vi "SR Doppler.vi"() -> ()   [LabVIEW 2012]
uses:
  user.lib/SpectralRadar.llb/Scan Pattern.lvclass
  user.lib/SpectralRadar.llb/Probe.lvclass
  user.lib/SpectralRadar.llb/Coloring.lvclass
  user.lib/SpectralRadar.llb/Colorscheme Selection.ctl
  user.lib/SpectralRadar.llb/Doppler Flag.ctl
  user.lib/SpectralRadar.llb/Coloring Byteorder.ctl
  <vilib>/Utility/error.llb/DialogType.ctl
  user.lib/SpectralRadar.llb/Calibration Selection.ctl
  user.lib/SpectralRadar.llb/Probe Parameter Int Selection.ctl
  user.lib/SpectralRadar.llb/Processing Parameter Int Selection.ctl
  user.lib/SpectralRadar.llb/Doppler Property Int.ctl
  user.lib/SpectralRadar.llb/set Complex Scan Output.vi
  user.lib/SpectralRadar.llb/display Data 2D.vi
  user.lib/SpectralRadar.llb/Doppler Processing.lvclass
  user.lib/SpectralRadar.llb/LabVIEW Helper.lvlib
  user.lib/SpectralRadar.llb/OCT Device.lvclass
  user.lib/SpectralRadar.llb/Processing.lvclass
  user.lib/SpectralRadar.llb/FullRange.lvclass
  user.lib/SpectralRadar.llb/Settings.lvclass
  user.lib/SpectralRadar.llb/FileSelection.lvlib
  user.lib/SpectralRadar.llb/Raw Data.lvclass
  user.lib/SpectralRadar.llb/Data.lvclass
  user.lib/SpectralRadar.llb/Colored Data.lvclass
  user.lib/SpectralRadar.llb/Complex Data.lvclass
panel:
  in  "Averaging Z":i32=1 min=1 max=20 step=1
  in  "Averaging X":i32=2 min=2 max=20 step=1
  out "Phase Graph":dbl[][](graph)
  out "Amplitude Graph":dbl[][](graph)
  in  "Absolute Phase Threshold":sgl=0.2
  in  "Signal Threshold [dB]":sgl
  out "Coloring":refnum<class "Coloring.lvclass">
  out "GalvoControl":refnum<class "Probe.lvclass">
  out "Scan Pattern":refnum<class "Scan Pattern.lvclass">
  out "AutoSafe":bool
  in  "Binning":i32(slide)=1 caption="Quality" min=1 max=200 step=1 scale=1.0..200.0
  in  "Options":bool
  in  "Window":T1(ring)
  in  "Palette":T2(ring)
  in  "ShowVideoImage":bool caption="Show Video Image"
  out "StreamingPath":path
  out "Image":T3(plugin-control)
  out "Frame Rate":dbl=6.134969234466553 format="%#_3g"
  in  "RunMeasurement":bool
  out "StopIndicator":bool
  in  "Brightness":sgl(slide)=0.5272727 caption="Sharpness" min=0 max=1 step=0.01 scale=0.0..1.0
  in  "Contrast":sgl(slide)=0.53333336 caption="Sharpness" min=0 max=1 step=0.01 scale=0.0..1.0
  in  "Saturation":sgl(slide)=0.5212121 caption="Sharpness" min=0 max=1 step=0.01 scale=0.0..1.0
  out "Spacing Z":dbl=2.0 min=1.0 max=500.0 step=1.0 format="%-#2_3f"
  in  "LowerBScanBorder":dbl=0.972000002861023 min=0.75 max=5.12 step=0.1 format="%.2f"
  in  "UpperBScanBorder":dbl min=0.0 max=0.5 step=0.10000000149011612 format="%.2f"
  out "Reference Intensity":sgl(slide) max=140000 scale=0.0..1.0
  out "Next File Name":path=path "D:/OCTData"
  in  "Set Path":bool
  in  "Recallibrate":bool
  in  "Range X [mm]":dbl=2.0 caption="Bereich [mm]" min=0.0 max=10.0 step=0.5 format="%_3f"
  out "Spacing X [µm]":dbl=2.0 min=1.0 max=500.0 step=1.0 format="%#_3g"
  in  "Columns":i32=1000 min=50 max=2500 step=1
  in  "Index of Refraction":dbl=1.0 min=1.0 max=5.0 step=0.10000000149011612 format="%.3f"
  in  "QuitApp":bool
  in  "Boundries":cluster{sgl, sgl}(slide)={76.65738, 42.00557} scale=-20.0..150.0
  out "B-Scan":sgl[][](graph)
  # "Version 5.1"
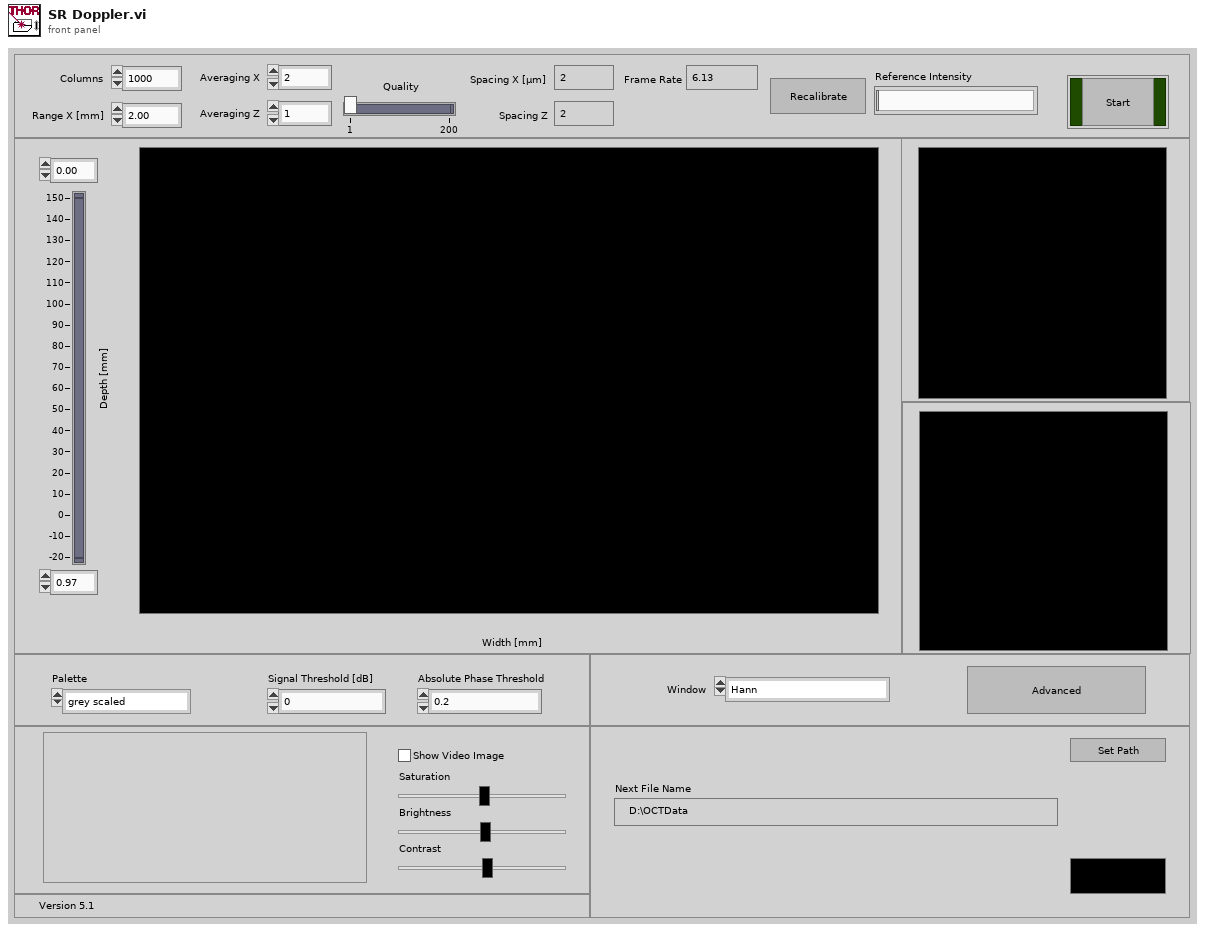
[diagram p1: front panel]
types:
  T1 = enum16{"Hann", "Hamming", "Gauss", "Tapered Cosine", "Blackman", "4 Term B-Harris"}
  T2 = enum16{"grey scaled", "grey scaled (inverted)", "color coded", "orange-black", "red-black"}
  T3 = typedef "IMAQ Image.ctl" = refnum<image>
  T4 = typedef "Coloring.lvclass/Coloring Byteorder.ctl" = enum16{"RGBA32", "BGRA32", "ARGB32", ""}
  T5 = typedef "Doppler Processing.lvclass/Doppler Flag.ctl" = enum16{"Doppler Velocity Scaling"}
  T6 = typedef "Coloring.lvclass/Colorscheme Selection.ctl" = enum16{"Black And White", "Inverted Black And White", "Color", "Black and Orange", "Black and Red", "Doppler Phase Coloring"}
  T7 = enum16{"Full Well Capacity", "z Spacing", "z Range", "Dynamc Range Min [dB]", "Dynamic Range Low [dB]", "Dynamic Range High [dB]", "Dynamic Range Max [dB]"}
  T8 = typedef "Processing.lvclass/Calibration Selection.ctl" = enum16{"Offset Errors", "Apodization Spectrum", "Apodization Vector", "Dispersion", "Chirp", "Extended Adjust", "Fixed Pattern"}
  T9 = typedef "Processing.lvclass/Processing Parameter Int Selection.ctl" = enum32{"Spectrum Averaging", "A-Scan Averaging", "B-Scan Averaging", "Zero Padding", "Number of Threads", "Fourier Averaging"}
  T10 = typedef "Probe.lvclass/Probe Parameter Int Selection.ctl" = enum16{"Apodization Cycles", "Oversampling", "Oversampling Slow Axis", "Speckle Reduction"}
  T11 = typedef "Doppler Processing.lvclass/Doppler Property Int.ctl" = enum16{"Doppler Averaging 1", "Doppler Averaging 2"}
  T12 = enum16{"Asynchronous Continuous", "Asynchronous Finite", "Synchronous"}
  T13 = typedef "Image Type" = u32
  T14 = typedef "DialogType.ctl" = u16
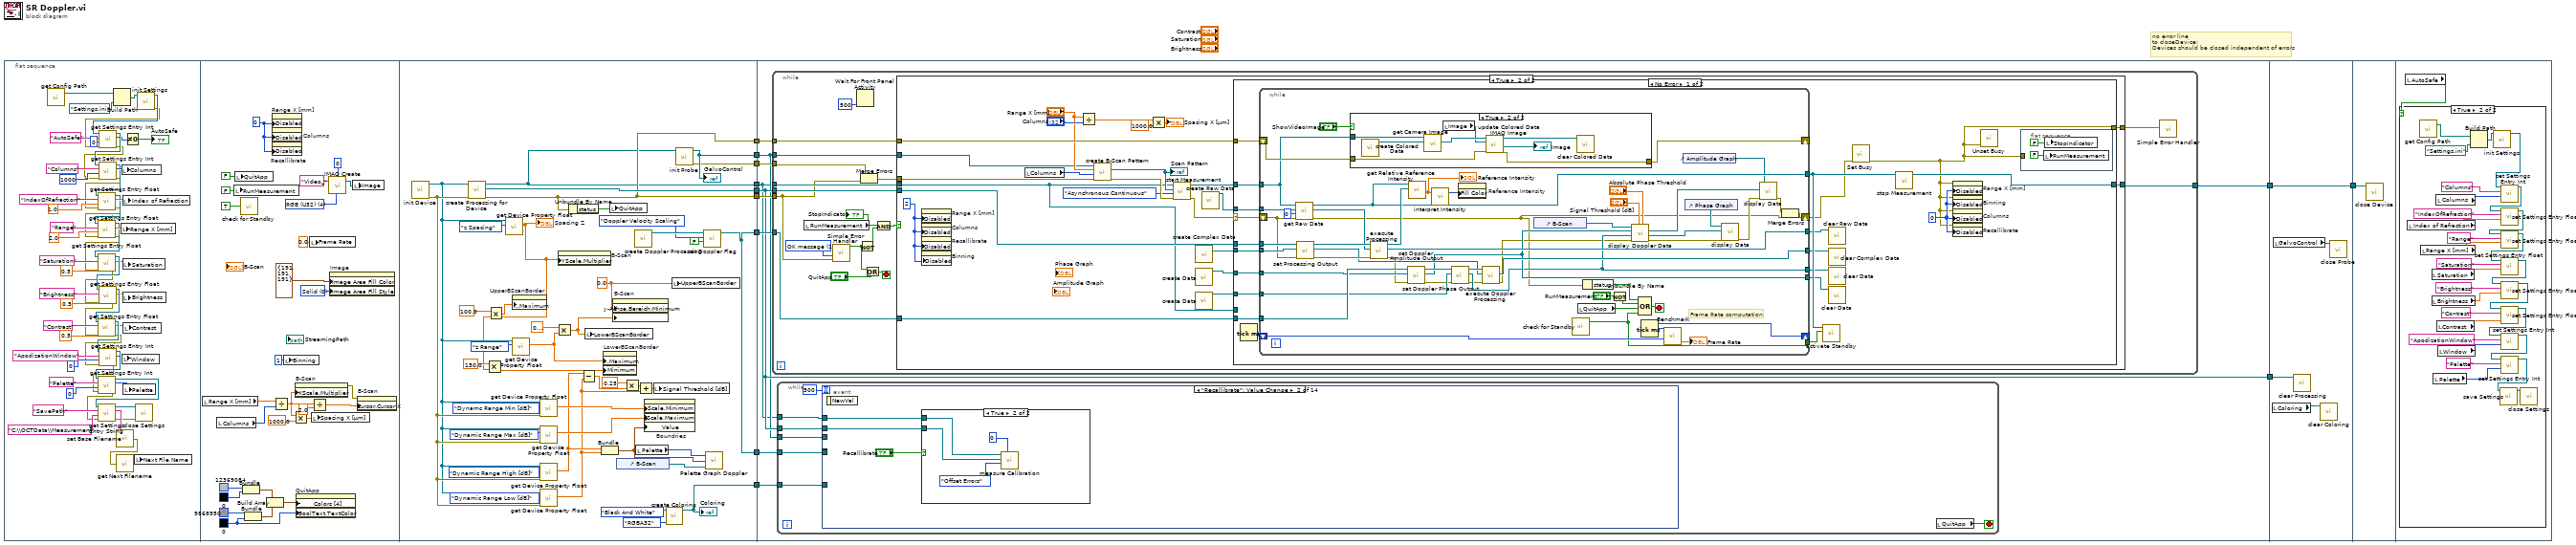
[diagram p0: block diagram]
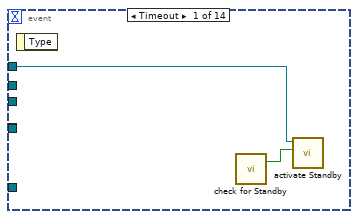
[diagram p2: hidden frame]
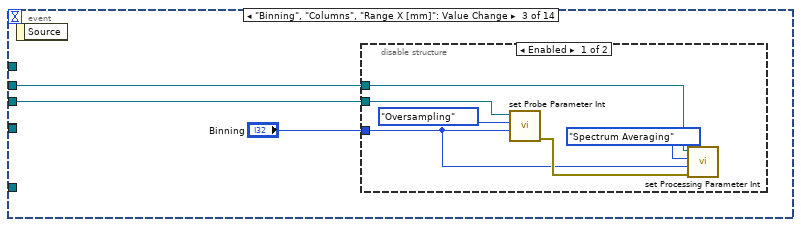
[diagram p4: hidden frame]
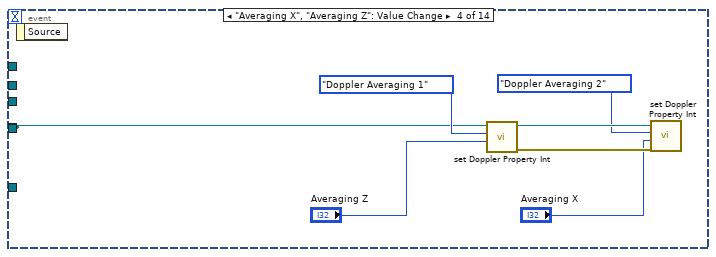
[diagram p6: hidden frame]
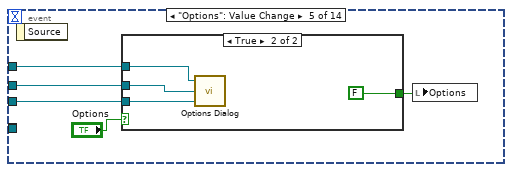
[diagram p7: hidden frame]
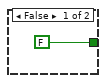
[diagram p8: hidden frame]
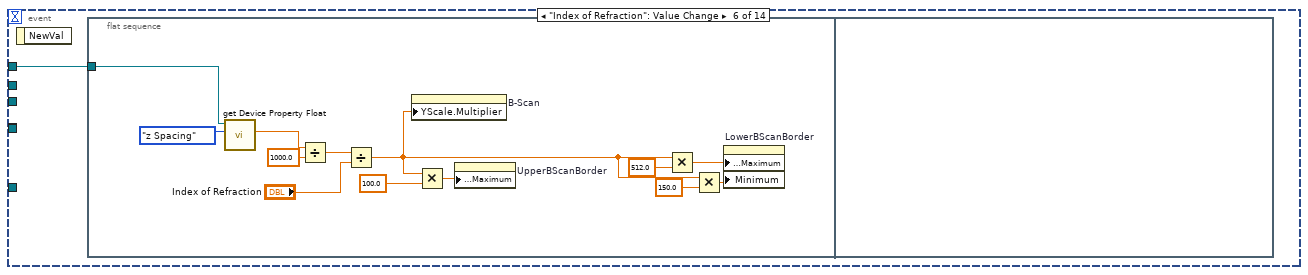
[diagram p9: hidden frame]
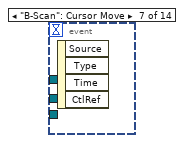
[diagram p10: hidden frame]
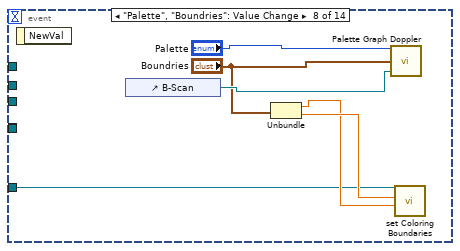
[diagram p11: hidden frame]
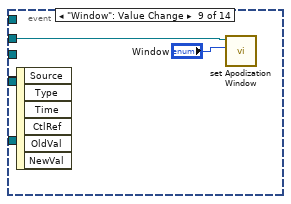
[diagram p12: hidden frame]
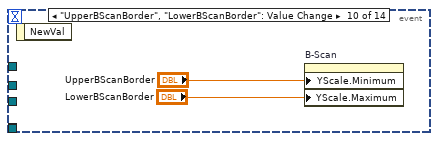
[diagram p13: hidden frame]
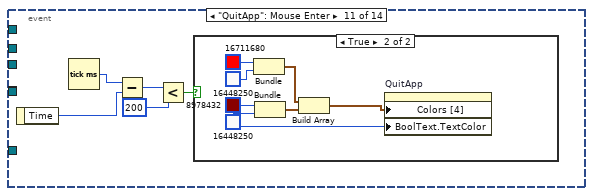
[diagram p14: hidden frame]
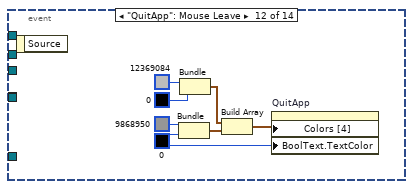
[diagram p16: hidden frame]
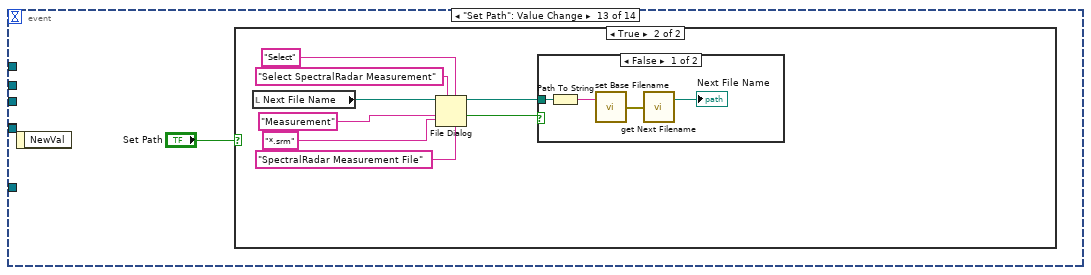
[diagram p17: hidden frame]
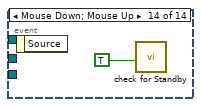
[diagram p20: hidden frame]
diagram:
  # "no error line\nto closeDevice:\nDevices should be closed independent of errors"
  n1 = flat-sequence {
    tunnel: [w109] -> w12
    tunnel: [w116] -> w9
    tunnel: [w128] -> w8
    tunnel: [w131] -> w6
    tunnel: [w116] -> w5
    tunnel: [w129] -> w4
    tunnel: [w113] -> w3
    tunnel: [w101] -> w2
    tunnel: [w101] -> w1
    tunnel: w12 -> [w141]
    tunnel: [w148] -> w10
    tunnel: w9 -> [w147]
    tunnel: w8 -> [w143]
    tunnel: [w143] -> w7
    tunnel: w6 -> [w142]
    tunnel: w5 -> [w146]
    tunnel: w4 -> [w145]
    tunnel: w3 -> [w139]
    tunnel: w2 -> [w144]
    tunnel: w1 -> [w140]
    tunnel: [w382] -> w11
    tunnel: w10 -> [w382]
    tunnel: w7 -> [w381]
    tunnel: w11 -> [w383]
    frame #0 {
      n2 = call "get Config Path.vi"() -> ("Path"=w24:path)  [unwired: 1 in, 1 out]
      n3 = Build Path(base path=w24, name or relative path=path "Settings.ini" ("Relative \"SpectralRadar.ini\" Path")) -> (appended path=w69:path)
      n4 = call "init Settings.vi"("Path to settings file"=w69) -> ("error out"=w23:errorcluster, "Settings"=w56:refnum<class "Settings.lvclass">)  [unwired: 5 in]
      n5 = call "get Settings Entry Int.vi"("error in (no error)"=w23, "Default Value"=0, "Node Name"="AutoSafe", "Settings"=w56) -> ("error out"=w21:errorcluster, "Value"=w53:i32, "Settings"=w57:refnum<class "Settings.lvclass">)  [unwired: 1 in]
      n6 = call "get Settings Entry Int.vi"("error in (no error)"=w21, "Default Value"=1000, "Node Name"="Columns", "Settings"=w57) -> ("error out"=w20:errorcluster, "Value"=w67:i32, "Settings"=w59:refnum<class "Settings.lvclass">)  [unwired: 1 in]
      n7 = call "get Settings Entry Float.vi"("error in (no error)"=w20, "Default Value"=1.0, "Node Name"="IndexOfRefraction", "Settings"=w59) -> ("error out"=w19:errorcluster, "Value"=w63:dbl, "Settings"=w58:refnum<class "Settings.lvclass">)  [unwired: 1 in]
      n8 = call "get Settings Entry Float.vi"("error in (no error)"=w19, "Default Value"=2.0, "Node Name"="Range", "Settings"=w58) -> ("error out"=w18:errorcluster, "Value"=w60:dbl, "Settings"=w49:refnum<class "Settings.lvclass">)  [unwired: 1 in]
      n9 = call "get Settings Entry Float.vi"("error in (no error)"=w18, "Default Value"=0.5, "Node Name"="Saturation", "Settings"=w49) -> ("error out"=w17:errorcluster, "Value"=w34:dbl, "Settings"=w46:refnum<class "Settings.lvclass">)  [unwired: 1 in]
      n10 = call "get Settings Entry Float.vi"("error in (no error)"=w17, "Default Value"=0.5, "Node Name"="Brightness", "Settings"=w46) -> ("error out"=w16:errorcluster, "Value"=w33:dbl, "Settings"=w39:refnum<class "Settings.lvclass">)  [unwired: 1 in]
      n11 = call "get Settings Entry Float.vi"("error in (no error)"=w16, "Default Value"=0.5, "Node Name"="Contrast", "Settings"=w39) -> ("error out"=w15:errorcluster, "Value"=w32:dbl, "Settings"=w38:refnum<class "Settings.lvclass">)  [unwired: 1 in]
      n12 = call "get Settings Entry Int.vi"("error in (no error)"=w15, "Default Value"=0, "Node Name"="ApodizationWindow", "Settings"=w38) -> ("error out"=w14:errorcluster, "Value"=w36:i32, "Settings"=w37:refnum<class "Settings.lvclass">)  [unwired: 1 in]
      n13 = call "get Settings Entry Int.vi"("error in (no error)"=w14, "Default Value"=0, "Node Name"="Palette", "Settings"=w37) -> ("error out"=w13:errorcluster, "Value"=w35:i32, "Settings"=w30:refnum<class "Settings.lvclass">)  [unwired: 1 in]
      n14 = call "get Settings Entry String.vi"("error in (no error)"=w13, "Default Value"="C:\\OCTData\\Measurement", "Node Name"="SavePath", "Settings"=w30) -> ("error out"=w22:errorcluster, "Value"=w27:string, "Settings"=w29:refnum<class "Settings.lvclass">)  [unwired: 1 in]
      n15 = call "set Base Filename.vi"("Base"=w27) -> ("error out"=w26:errorcluster)  [unwired: 1 in]
      n16 = call "get Next Filename.vi"("error in (no error)"=w26) -> ("Next File Name"=w25:path)  [unwired: 1 out]
      n17 = local write "Range X [mm]"(w60) -> ()
      n18 = local write "Columns"(w67) -> ()
      n19 = local write "Window"(w36) -> ()
      n20 = local write "Index of Refraction"(w63) -> ()
      n21 = local write "Saturation"(w34) -> ()
      n22 = local write "Brightness"(w33) -> ()
      n23 = local write "Contrast"(w32) -> ()
      n24 = local write "Palette"(w35) -> ()
      n25 = Not Equal To 0?(x=w53) -> (x != 0?=→"AutoSafe":bool)
      n26 = local write "Next File Name"(w25) -> ()
      n27 = call "close Settings.vi"("error in (no error)"=w22, "Settings"=w29) -> ()  [unwired: 5 in, 1 out]
    }
    frame #1 {
      w73 = T13 4 items=["Grayscale (U8)", "Grayscale (I16)", "Grayscale (SGL)", "Complex (CSG)", "RGB (U32)", "HSL (U32)", "RGB (U64)", "Grayscale (U16)"] ("Image Type")
      w78 = u32 0 items=["Default"=3, "Solid"=0, "Hatch"=2] ("Image Area:Background:Fill Style")
      w93 = u32 0
      w97 = u8 0 ("Deaktiviert")
      n28 = local read "Range X [mm]"() -> (w85:dbl)
      n29 = local read "Columns"() -> (w80:i32)
      n30 = local write "RunMeasurement"(FALSE ("s/t")) -> ()
      n31 = local write "QuitApp"(FALSE ("QuitApp")) -> ()
      n32 = call "check for Standby.vi"("ResetTimer"=TRUE) -> ()  [unwired: 2 out]
      n33 = Bundle(u32 12369084, u32 0) -> (w90:cluster{u32, u32})  [unwired: 1 in]
      n34 = Bundle(u32 9868950, w93) -> (w91:cluster{u32, u32})  [unwired: 1 in]
      n35 = Build Array(w90, w91) -> (w92:cluster{u32, u32}[])
      n36 = property on="Range X [mm]" class="DigNum (strict)"("Disabled"=w97) -> ()  [unwired: 2 in, 2 out]
      n37 = property on="Columns" class="DigNum (strict)"("Disabled"=w97) -> ()  [unwired: 2 in, 2 out]
      n38 = property on="Recallibrate" class="Bool"("Disabled"=w97) -> ()  [unwired: 2 in, 2 out]
      n39 = Divide(x=w85, y=w80) -> (x/y=w83:dbl)
      n40 = local write "Binning"(1 ("Binning")) -> ()
      n41 = Multiply(x=w83, y=1000.0) -> (x*y=w81:dbl)
      n42 = property on="B-Scan" class="IntGraph (strict)"("XScale.Multiplier"=w83) -> (error out=w86:errorcluster)  [unwired: 2 in, 1 out]
      n43 = property on="QuitApp" class="Bool (strict)"("Colors [4]"=w92, "BoolText.TextColor"=w93) -> ()  [unwired: 2 in, 2 out]
      n44 = local write "Frame Rate"(0.0 ("Frame Rate")) -> ()
      n45 = Divide(x=w83, y=2.0) -> (x/y=w82:dbl)
      n46 = local write "Spacing X [µm]"(w81) -> ()
      n47 = call "IMAQ Create"("Border Size"=0, "Image Name"="Video_", "Image Type"=w73) -> ("New Image"=w71:T3)  [unwired: 2 in, 1 out]
      n48 = property on="Image" class="ImageControl"("Image Area Fill Color"=cluster{"Red":u8, "Green":u8, "Blue":u8} {"Red"=191, "Green"=191, "Blue"=191} ("Image Area:Background:Fill Color"), "Image Area Fill Style"=w78) -> ()  [unwired: 2 in, 2 out]
      n49 = local write "Image"(w71) -> ()
      n50 = property on="B-Scan" class="IntGraph (strict)"(error in=w86, "Cursor.Cursor X"=w82) -> ()  [unwired: 1 in, 2 out]
    }
    frame #2 {
      w133 = 0.0 ("y")
      n51 = call "init Device.vi"() -> ("error out"=w127:errorcluster, "OCTDevice"=w120:refnum<class "OCT Device.lvclass">)  [unwired: 6 in]
      n52 = call "create Processing for Device.vi"("error in (no error)"=w127, "OCTDevice"=w120) -> ("error out"=w116:errorcluster, "Processing"=w128:refnum<class "Processing.lvclass">, "OCTDevice"=w109:refnum<class "OCT Device.lvclass">)  [unwired: 3 in]
      n53 = call "get Device Property Float.vi"("Device Property Float Selection"=T7."z Spacing", "OCTDevice"=w120) -> ("Value"=w115:dbl)  [unwired: 3 in, 2 out]
      "Spacing Z" <- w115
      n54 = Multiply(x=150.0, y=w115) -> (x*y=w135:dbl)
      n55 = Multiply(x=100.0, y=w115) -> (x*y=w138:dbl)
      n56 = property on="UpperBScanBorder" class="DigNum (strict)"("Wertebereich:Maximum"=w138) -> ()  [unwired: 2 in, 2 out]
      n57 = call "get Device Property Float.vi"("Device Property Float Selection"=T7."z Range", "OCTDevice"=w120) -> ("Value"=w118:dbl)  [unwired: 3 in, 2 out]
      n58 = call "get Device Property Float.vi"("error in (no error)"=w127, "Device Property Float Selection"=T7."Dynamc Range Min [dB]", "OCTDevice"=w120) -> ("Value"=w126:dbl)  [unwired: 2 in, 2 out]
      n59 = call "get Device Property Float.vi"("error in (no error)"=w127, "Device Property Float Selection"=T7."Dynamic Range Max [dB]", "OCTDevice"=w120) -> ("Value"=w125:dbl)  [unwired: 2 in, 2 out]
      n60 = call "get Device Property Float.vi"("error in (no error)"=w127, "Device Property Float Selection"=T7."Dynamic Range High [dB]", "OCTDevice"=w120) -> ("Value"=w107:dbl)  [unwired: 2 in, 2 out]
      n61 = call "get Device Property Float.vi"("error in (no error)"=w127, "Device Property Float Selection"=T7."Dynamic Range Low [dB]", "OCTDevice"=w120) -> ("Value"=w106:dbl)  [unwired: 2 in, 2 out]
      n62 = Multiply(x=0.800000011920929, y=w118) -> (x*y=w132:dbl)
      n63 = property on="B-Scan" class="IntGraph (strict)"("YScale.Multiplier"=w115) -> ()  [unwired: 2 in, 2 out]
      n64 = Unbundle By Name(w116) -> ("status"=w130:bool)
      n65 = Subtract(x=w107, y=w106) -> (x-y=w104:dbl)
      n66 = local write "LowerBScanBorder"(w132) -> ()
      n67 = Bundle("Value"=w107, "Value"=w106) -> (w112:cluster{"Value":dbl, "Value":dbl})  [unwired: 1 in]
      n68 = property on="LowerBScanBorder" class="DigNum (strict)"("Wertebereich:Maximum"=w118, "Minimum"=w135) -> ()  [unwired: 2 in, 2 out]
      n69 = local write "QuitApp"(w130) -> ()
      n70 = property on="B-Scan" class="IntGraph (strict)"("y-Achse.Bereich:Minimum"=w133, "y-Achse.Bereich:Maximum"=w132) -> ()  [unwired: 2 in, 2 out]
      n71 = control-ref of="B-Scan"() -> (w110:refnum<vi>)
      n72 = Multiply(x=0.25, y=w104) -> (x*y=w105:dbl)
      n73 = call "create Doppler Processing.vi"() -> ("Doppler Processing"=w102:refnum<class "Doppler Processing.lvclass">)  [unwired: 6 in, 1 out]
      n74 = local read "Palette"() -> (w111:T2)
      n75 = Add(x=w105, y=w106) -> (x+y=w108:dbl)
      n76 = property on="Boundries" class="Slide (strict)"("Scale.Minimum"=w126, "Scale.Maximum"=w125, "Value"=w112) -> ()  [unwired: 2 in, 2 out]
      n77 = local write "Signal Threshold [dB]"(w108) -> ()
      n78 = call "create Coloring.vi"("Color Byte Order"=Coloring_Byteorder."RGBA32", "Color Table Selection"=Colorscheme_Selection."Black And White") -> ("Coloring"=w113:refnum<class "Coloring.lvclass">)  [unwired: 4 in, 1 out]
      "Coloring" <- w113
      n79 = local write "UpperBScanBorder"(w133) -> ()
      n80 = call "init Probe.vi"("OCT Device"=w109) -> ("error out"=w129:errorcluster, "GalvoControl"=w131:refnum<class "Probe.lvclass">)  [unwired: 5 in]
      "GalvoControl" <- w131
      n81 = call "set Doppler Flag.vi"("Boolean"=FALSE, "Doppler Flag"=Doppler_Flag."Doppler Velocity Scaling", "DopplerProcessing in"=w102) -> ("DopplerProcessing out"=w101:refnum<class "Doppler Processing.lvclass">)  [unwired: 3 in, 1 out]
      n82 = call "Palette Graph Doppler.vi"("Reference to the B-scan Graph"=w110, "Boundaries"=w112, "Palette"=w111) -> ()
    }
    frame #3 {
      n83 = while {
        tunnel: w141 -> [w261]
        tunnel: [w260] -> w148
        tunnel: w147 -> [w259]
        tunnel: w143 -> [w258]
        tunnel: w142 -> [w257]
        tunnel: w146 -> [w256]
        tunnel: w145 -> [w250]
        tunnel: w144 -> [w248]
        stop <- w263 stop-if-true
        w249 = T14 1 items=["no dialog", "OK message", "continue or stop message", "OK message + warnings", "continue/stop + warnings"] ("type of dialog (OK msg:1)")
        n84 = local read "RunMeasurement"() -> (w254:bool)
        "StopIndicator" <- w254
        n85 = call <vilib>:"Simple Error Handler.vi"("type of dialog (OK msg:1)"=w249, "error in (no error)"=w256) -> ("error?"=w253:bool)  [unwired: 3 in, 4 out]
        n86 = Wait For Front Panel Activity(1:500 ("Timeout in ms (-1 kein Timeout)")) -> ()  [unwired: 2 in, 1 out]
        n87 = Not(x=w253) -> (.not. x?=w252:bool)
        n88 = Merge Errors(w250, w256) -> (w251:errorcluster)
        n89 = Or(x=w253, y="QuitApp") -> (x .or. y?=w263:bool)
        n90 = And(x=w254, y=w252) -> (x .and. y?=w255:bool)
        n91 = case shown="True" w255 {
          tunnel: [w267 w291] -> w265
          tunnel: w251 -> [w267 w268]
          tunnel: w261 -> [w266 w274]
          tunnel: [w266 w285] -> w260
          tunnel: w259 -> [_ w284]
          tunnel: w258 -> [_ w278]
          tunnel: w257 -> [_ w280]
          tunnel: w248 -> [_ w269]
          frame False {
          }
          frame True {
            w279 = u8 2 ("Deaktiviert")
            n92 = property on="Range X [mm]" class="DigNum (strict)"("Disabled"=w279) -> ()  [unwired: 2 in, 2 out]
            n93 = property on="Columns" class="DigNum (strict)"("Disabled"=w279) -> ()  [unwired: 2 in, 2 out]
            n94 = property on="Recallibrate" class="Bool"("Disabled"=w279) -> ()  [unwired: 2 in, 2 out]
            n95 = property on="Binning" class="Slide (strict)"("Disabled"=w279) -> ()  [unwired: 2 in, 2 out]
            n96 = local read "Columns"() -> (w282:i32)
            n97 = Divide(x="Range X [mm]", y="Columns") -> (x/y=w289:dbl)
            n98 = call "create B-Scan Pattern.vi"("error in (no error)"=w268, "AScans"=w282, "Range"="Range X [mm]", "Probe"=w280) -> ("error out"=w281:errorcluster, "Scan Pattern"=w277:refnum<class "Scan Pattern.lvclass">)  [unwired: 2 in, 1 out]
            "Scan Pattern" <- w277
            n99 = Multiply(x=w289, y=1000.0) -> (x*y=→"Spacing X [µm]":dbl)
            n100 = call "start Measurement.vi"("error in (no error)"=w281, "Acquisition Type"=T12."Asynchronous Continuous", "Scan Pattern"=w277, "OCTDevice"=w274) -> ("error out"=w275:errorcluster, "OCTDevice"=w290:refnum<class "OCT Device.lvclass">)  [unwired: 1 in, 1 out]
            n101 = call "create Data.vi"() -> ("Data"=w271:refnum<class "Data.lvclass">)  [unwired: 6 in, 1 out]
            n102 = call "create Data.vi"() -> ("Data"=w270:refnum<class "Data.lvclass">)  [unwired: 6 in, 1 out]
            n103 = call "create Complex Data.vi"() -> ("Complex Data"=w272:refnum<class "Complex Data.lvclass">)  [unwired: 2 in, 1 out]
            n104 = call "create Raw Data.vi"() -> ("Raw Data"=w276:refnum<class "Raw Data.lvclass">)  [unwired: 6 in, 1 out]
            n105 = case shown="No Error" w275 {
              selector: w275 -> [w302 w378]
              tunnel: [w303 _] -> w291
              tunnel: w284 -> [w311 _]
              tunnel: w290 -> [w310 w375]
              tunnel: [w309 w374] -> w285
              tunnel: w278 -> [w305 _]
              tunnel: w276 -> [w301 _]
              tunnel: w274 -> [_ _]
              tunnel: w272 -> [w298 _]
              tunnel: w271 -> [w297 _]
              tunnel: w270 -> [w296 _]
              tunnel: w269 -> [w295 _]
              frame No Error {
                w304 = u8 0 ("Deaktiviert")
                n106 = Tick Count (ms)() -> (millisecond timer value=w307:u32)
                n107 = while {
                  shift-right: [w362] -> _
                  shift-left: w307 -> [w360]
                  tunnel: w310 -> [w353]
                  tunnel: [w351] -> w306
                  tunnel: [w335] -> w308
                  tunnel: w305 -> [w349]
                  shift-right: [w354] -> _
                  shift-left: w311 -> [w364]
                  shift-right: [w318] -> w300
                  shift-left: w302 -> [w321]
                  tunnel: w301 -> [w352]
                  tunnel: [w343] -> w299
                  tunnel: w298 -> [w342]
                  tunnel: w297 -> [w340]
                  tunnel: w296 -> [w338]
                  tunnel: w295 -> [w341]
                  tunnel: [w331] -> w294
                  tunnel: [w332] -> w293
                  tunnel: [w334] -> w292
                  stop <- w358 stop-if-true
                  # "Frame Rate computation"
                  n108 = call "get Raw Data.vi"("error in (no error)"=w321, "Camera Index"=0, "RawData in"=w352, "OCTDevice in"=w353) -> ("error out"=w319:errorcluster, "RawData out"=w347:refnum<class "Raw Data.lvclass">, "OCTDevice out"=w335:refnum<class "OCT Device.lvclass">)  [unwired: 1 in]
                  n109 = call-poly "set Processing Output.vi"("error in (no error)"=w321, "Complex Data in"=w342, "Processing"=w349) -> ("error out"=w346:errorcluster, "Complex Data out"=w336:refnum<class "Complex Data.lvclass">, "Processing"=w348:refnum<class "Processing.lvclass">)  [unwired: 2 in]
                  n110 = case shown="True" "ShowVideoImage" {
                    tunnel: w353 -> [_ w373]
                    tunnel: w364 -> [w365 w370]
                    tunnel: [w365 w369] -> w354
                    frame False {
                    }
                    frame True {
                      n111 = call "create Colored Data.vi"() -> ("Colored Data"=w372:refnum<class "Colored Data.lvclass">)  [unwired: 6 in, 1 out]
                      n112 = call "get Camera Image.vi"("Colored Data in"=w372, "OCTDevice in"=w373) -> ("Colored Data out"=w371:refnum<class "Colored Data.lvclass">)  [unwired: 5 in, 2 out]
                      n113 = local read "Image"() -> (w367:T3)
                      n114 = call "update Colored Data IMAQ Image.vi"("error in (no error)"=w370, "Image in"=w367, "Colored Data"=w371) -> ("error out"=w369:errorcluster, "Image out"=→"Image":T3, "Colored Data"=w366:refnum<class "Colored Data.lvclass">)  [unwired: 2 in]
                      n115 = call "clear Colored Data.vi"("Colored Data"=w366) -> ()  [unwired: 6 in, 1 out]
                    }
                  }
                  n116 = call "execute Processing.vi"("error in (no error)"=w346, "Raw Data"=w347, "Processing"=w348) -> ("error out"=w317:errorcluster, "Raw Data"=w343:refnum<class "Raw Data.lvclass">, "Processing"=w345:refnum<class "Processing.lvclass">)  [unwired: 2 in]
                  n117 = call "set Doppler Amplitude Output.vi"("error in (no error)"=w317, "Data in"=w340, "DopplerProcessing in"=w341) -> ("error out"=w316:errorcluster, "Data out"=w332:refnum<class "Data.lvclass">, "DopplerProcessing out"=w339:refnum<class "Doppler Processing.lvclass">)  [unwired: 2 in]
                  n118 = call "get Relative Reference Intensity.vi"("Processing"=w345, "OCTDevice"=w335) -> ("Relative Reference Intensity"=w344:dbl)  [unwired: 2 in, 3 out]
                  "Reference Intensity" <- w344
                  n119 = call "interpret Intensity.vi"("Intensity"=w344) -> ("Color"=w356:u32)  [unwired: 1 in, 1 out]
                  n120 = call "set Doppler Phase Output.vi"("error in (no error)"=w316, "Data in"=w338, "DopplerProcessing in"=w339) -> ("error out"=w315:errorcluster, "Data out"=w331:refnum<class "Data.lvclass">, "DopplerProcessing out"=w337:refnum<class "Doppler Processing.lvclass">)  [unwired: 2 in]
                  n121 = property on="Reference Intensity" class="Slide (strict)"("Fill Color"=w356) -> ()  [unwired: 2 in, 2 out]
                  n122 = call "execute Doppler Processing.vi"("error in (no error)"=w315, "Complex Data in"=w336, "DopplerProcessing in"=w337) -> ("error out"=w330:errorcluster, "Complex Data out"=w334:refnum<class "Complex Data.lvclass">)  [unwired: 2 in, 1 out]
                  n123 = control-ref of="B-Scan"() -> (w333:refnum<vi>)
                  n124 = call "check for Standby.vi"() -> ("TimeOut"=w351:bool)  [unwired: 1 in, 1 out]
                  n125 = local read "QuitApp"() -> (w350:bool)
                  n126 = Unbundle By Name(w319) -> ("status"=w355:bool)
                  n127 = Not(x="RunMeasurement") -> (.not. x?=w359:bool)
                  n128 = call "display Doppler Data.vi"("Phase Threadshold"="Absolute Phase Threshold", "dB Threashold"="Signal Threshold [dB]", "error in (no error)"=w330, "Phase Data in"=w331, "Amp Data in"=w332, "IntGraph Refnum"=w333) -> ("error out"=w323:errorcluster, "Phase Data in"=w326:refnum<class "Data.lvclass">, "Amp Data in"=w327:refnum<class "Data.lvclass">)  [unwired: 1 in]
                  n129 = Compound Arithmetic op=OR(w355, w359, w350, w351) -> (w358:bool)
                  n130 = Tick Count (ms)() -> (millisecond timer value=w362:u32)
                  n131 = call "Benchmark.vi"("TimeStart"=w360, "TimeFinish"=w362) -> ("AverageFrameRate"=→"Frame Rate":sgl)  [unwired: 2 in, 2 out]
                  n132 = control-ref of="Amplitude Graph"() -> (w325:refnum<vi>)
                  n133 = control-ref of="Phase Graph"() -> (w324:refnum<vi>)
                  n134 = call-poly "display Data.vi"("error in (no error)"=w323, "Data in"=w326, "IntGraph Refnum"=w324) -> ("error out"=w322:errorcluster)  [unwired: 2 in, 2 out]
                  n135 = call-poly "display Data.vi"("error in (no error)"=w322, "Data in"=w327, "IntGraph Refnum"=w325) -> ("error out"=w320:errorcluster)  [unwired: 2 in, 2 out]
                  n136 = Merge Errors(w320, w319) -> (w318:errorcluster)
                }
                n137 = call "activate Standby.vi"("StandBy"=w306, "OCTDevice"=w308) -> ()  [unwired: 4 in, 2 out]
                n138 = call "clear Raw Data.vi"("Raw Data"=w299) -> ()  [unwired: 6 in, 1 out]
                n139 = call "clear Complex Data.vi"("Complex Data"=w292) -> ()  [unwired: 6 in, 1 out]
                n140 = call "clear Data.vi"("Data"=w294) -> ()  [unwired: 6 in, 1 out]
                n141 = call "clear Data.vi"("Data"=w293) -> ()  [unwired: 6 in, 1 out]
                n142 = call <vilib>:"Set Busy.vi"("error in (no error)"=w300) -> ("error out"=w303:errorcluster)  [unwired: 9 in, 1 out]
                n143 = call "stop Measurement.vi"("OCTDevice"=w308) -> ("OCTDevice"=w309:refnum<class "OCT Device.lvclass">)  [unwired: 5 in, 1 out]
                n144 = property on="Range X [mm]" class="DigNum (strict)"(error in=w303, "Disabled"=w304) -> ()  [unwired: 1 in, 2 out]
                n145 = property on="Binning" class="Slide (strict)"(error in=w303, "Disabled"=w304) -> ()  [unwired: 1 in, 2 out]
                n146 = property on="Columns" class="DigNum (strict)"(error in=w303, "Disabled"=w304) -> ()  [unwired: 1 in, 2 out]
                n147 = property on="Recallibrate" class="Bool"(error in=w303, "Disabled"=w304) -> ()  [unwired: 1 in, 2 out]
                n148 = call <vilib>:"Unset Busy.vi"("error in (no error)"=w303) -> ()  [unwired: 10 in, 1 out]
                n149 = flat-sequence {
                  tunnel: w303 -> [_]
                  frame #0 {
                    n150 = local write "RunMeasurement"(FALSE ("StopIndicator")) -> ()
                    n151 = local write "StopIndicator"(FALSE ("StopIndicator")) -> ()
                  }
                }
              }
              frame Error {
                w377 = T14 1 items=["no dialog", "OK message", "continue or stop message", "OK message + warnings", "continue/stop + warnings"] ("type of dialog (OK msg:1)")
                w376 = FALSE ("RunMeasurement")
                n152 = call <vilib>:"Simple Error Handler.vi"("type of dialog (OK msg:1)"=w377, "error in (no error)"=w378) -> ()  [unwired: 3 in, 5 out]
                n153 = local write "RunMeasurement"(w376) -> ()
                n154 = local write "StopIndicator"(w376) -> ()
                n155 = call "stop Measurement.vi"("OCTDevice"=w375) -> ("OCTDevice"=w374:refnum<class "OCT Device.lvclass">)  [unwired: 5 in, 1 out]
              }
            }
          }
        }
        n156 = call <vilib>:"Simple Error Handler.vi"("error in (no error)"=w265) -> ()  [unwired: 4 in, 5 out]
      }
      n157 = while {
        tunnel: w143 -> [w154]
        tunnel: w142 -> [w153]
        tunnel: w141 -> [w152]
        tunnel: w140 -> [w151]
        tunnel: w139 -> [w150]
        stop <- w155 stop-if-true
        n158 = event shown="[1] \"Recallibrate\": Value Change" {
          selector: _ -> [_ _ _ _ _ _ _ _ _ _ _ _ _ _]
          dyn-events: _ -> [_ _ _ _ _ _ _ _ _ _ _ _ _ _]
          timeout: 500 ("Timeout in ms (-1 kein Timeout)") -> [_ _ _ _ _ _ _ _ _ _ _ _ _ _]
          tunnel: w154 -> [_ w158 w165 _ w182 _ _ _ w211 _ _ _ _ _]
          tunnel: w153 -> [_ _ w166 _ w181 _ _ _ _ _ _ _ _ _]
          tunnel: w152 -> [w156 w159 _ _ w183 w191 _ _ _ _ _ _ _ _]
          tunnel: [_ _ _ w174 _ _ _ _ _ _ _ _ _ _] -> _
          tunnel: w151 -> [_ _ _ w174 _ _ _ _ _ _ _ _ _ _]
          tunnel: w150 -> [_ _ _ _ _ _ _ w205 _ _ _ _ _ _]
          event Timeout {
            n159 = event-data() -> ()  [unwired: 1 in, 1 out]
            n160 = call "check for Standby.vi"() -> ("TimeOut"=w157:bool)  [unwired: 1 in, 1 out]
            n161 = call "activate Standby.vi"("StandBy"=w157, "OCTDevice"=w156) -> ()  [unwired: 4 in, 2 out]
          }
          event "Recallibrate": Value Change {
            n162 = event-data() -> ()  [unwired: 1 in, 1 out]
            n163 = case shown="True" "Recallibrate" {
              tunnel: w159 -> [_ w163]
              tunnel: w158 -> [_ w162]
              frame False {
              }
              frame True {
                n164 = call "measure Calibration.vi"("Camera Index"=0, "Calibration Data"=Calibration_Selection."Offset Errors", "Processing"=w162, "OCTDevice"=w163) -> ()  [unwired: 2 in, 3 out]
              }
            }
          }
          event "Binning", "Columns", "Range X [mm]": Value Change {
            n165 = event-data() -> ()  [unwired: 1 in, 1 out]
            n166 = disable-structure shown="Enabled" {
              disable-tunnel: "Binning" -> [w168 _]
              disable-tunnel: w166 -> [w170 _]
              disable-tunnel: w165 -> [w169 _]
              frame Enabled {
                n167 = call "set Probe Parameter Int.vi"("Value"=w168, "Probe Parameter Int"=Probe_Parameter_Int_Selection."Oversampling", "GalvoControl"=w170) -> ("error out"=w172:errorcluster)  [unwired: 3 in, 1 out]
                n168 = call "set Processing Parameter Int.vi"("error in (no error)"=w172, "Value"=w168, "Processing Paramter Int Selection"=Processing_Parameter_Int_Selection."Spectrum Averaging", "Processing in"=w169) -> ()  [unwired: 2 in, 2 out]
              }
              frame Disabled {
              }
            }
          }
          event "Averaging X", "Averaging Z": Value Change {
            n169 = event-data() -> ()  [unwired: 1 in, 1 out]
            n170 = call "set Doppler Property Int.vi"("Value"="Averaging Z", "Doppler Property"=Doppler_Property_Int."Doppler Averaging 1", "DopplerProcessing in"=w174) -> ("error out"=w177:errorcluster, "DopplerProcessing out"=w178:refnum<class "Doppler Processing.lvclass">)  [unwired: 3 in]
            n171 = call "set Doppler Property Int.vi"("error in (no error)"=w177, "Value"="Averaging X", "Doppler Property"=Doppler_Property_Int."Doppler Averaging 2", "DopplerProcessing in"=w178) -> ()  [unwired: 2 in, 2 out]
          }
          event "Options": Value Change {
            n172 = event-data() -> ()  [unwired: 1 in, 1 out]
            n173 = case shown="True" "Options" {
              tunnel: [FALSE ("Options") FALSE ("Options")] -> w184
              tunnel: w183 -> [_ w189]
              tunnel: w182 -> [_ w188]
              tunnel: w181 -> [_ w187]
              frame False {
              }
              frame True {
                n174 = call "Options Dialog.vi"("GalvoControl"=w187, "Processing"=w188, "OCT Device"=w189) -> ()  [unwired: 1 in]
              }
            }
            n175 = local write "Options"(w184) -> ()
          }
          event "Index of Refraction": Value Change {
            n176 = event-data() -> ()  [unwired: 1 in, 1 out]
            n177 = flat-sequence {
              tunnel: w191 -> [w192]
              frame #0 {
                n178 = call "get Device Property Float.vi"("Device Property Float Selection"=T7."z Spacing", "OCTDevice"=w192) -> ("Value"=w194:dbl)  [unwired: 3 in, 2 out]
                n179 = Divide(x=w194, y=1000.0) -> (x/y=w203:dbl)
                n180 = Divide(x=w203, y="Index of Refraction") -> (x/y=w196:dbl)
                n181 = property on="B-Scan" class="IntGraph (strict)"("YScale.Multiplier"=w196) -> ()  [unwired: 2 in, 2 out]
                n182 = Multiply(x=w196, y=100.0) -> (x*y=w200:dbl)
                n183 = property on="UpperBScanBorder" class="DigNum (strict)"("Wertebereich:Maximum"=w200) -> ()  [unwired: 2 in, 2 out]
                n184 = Multiply(x=w196, y=512.0) -> (x*y=w199:dbl)
                n185 = Multiply(x=w196, y=150.0) -> (x*y=w197:dbl)
                n186 = property on="LowerBScanBorder" class="DigNum (strict)"("Wertebereich:Maximum"=w199, "Minimum"=w197) -> ()  [unwired: 2 in, 2 out]
              }
              frame #1 {
              }
            }
          }
          event "B-Scan": Cursor Move {
            n187 = event-data() -> ()  [unwired: 1 in, 4 out]
          }
          event "Palette", "Boundries": Value Change {
            n188 = event-data() -> ()  [unwired: 1 in, 1 out]
            n189 = control-ref of="B-Scan"() -> (w207:refnum<vi>)
            n190 = Unbundle("Boundries") -> (w209:sgl, w210:sgl)
            n191 = call "Palette Graph Doppler.vi"("Reference to the B-scan Graph"=w207, "Boundaries"="Boundries", "Palette"="Palette") -> ()
            n192 = call "set Coloring Boundaries.vi"("Danymic Range High [dB]"=w209, "Dynamic Range Low [dB]"=w210, "Coloring in"=w205) -> ()  [unwired: 3 in, 2 out]
          }
          event "Window": Value Change {
            n193 = event-data() -> ()  [unwired: 1 in, 6 out]
            n194 = call "set Apodization Window.vi"("Window"="Window", "Processing"=w211) -> ()  [unwired: 4 in, 2 out]
          }
          event "UpperBScanBorder", "LowerBScanBorder": Value Change {
            n195 = event-data() -> ()  [unwired: 1 in, 1 out]
            n196 = property on="B-Scan" class="IntGraph (strict)"("YScale.Minimum"="UpperBScanBorder", "YScale.Maximum"="LowerBScanBorder") -> ()  [unwired: 2 in, 2 out]
          }
          event "QuitApp": Mouse Enter {
            n197 = event-data() -> ("Time"=w218:u32)  [unwired: 1 in]
            n198 = Tick Count (ms)() -> (millisecond timer value=w219:u32)
            n199 = Subtract(x=w219, y=w218) -> (x-y=w217:u32)
            n200 = Less?(x=w217, y=u32 200) -> (x < y?=w215:bool)
            n201 = case shown="True" w215 {
              frame False {
              }
              frame True {
                w220 = u32 16448250
                n202 = Bundle(u32 16711680, u32 16448250) -> (w222:cluster{u32, u32})  [unwired: 1 in]
                n203 = Bundle(u32 8978432, w220) -> (w221:cluster{u32, u32})  [unwired: 1 in]
                n204 = Build Array(w222, w221) -> (w224:cluster{u32, u32}[])
                n205 = property on="QuitApp" class="Bool (strict)"("Colors [4]"=w224, "BoolText.TextColor"=w220) -> ()  [unwired: 2 in, 2 out]
              }
            }
          }
          event "QuitApp": Mouse Leave {
            w227 = u32 0
            n206 = event-data() -> ()  [unwired: 1 in, 1 out]
            n207 = Bundle(u32 9868950, w227) -> (w228:cluster{u32, u32})  [unwired: 1 in]
            n208 = Bundle(u32 12369084, u32 0) -> (w229:cluster{u32, u32})  [unwired: 1 in]
            n209 = Build Array(w229, w228) -> (w233:cluster{u32, u32}[])
            n210 = property on="QuitApp" class="Bool (strict)"("Colors [4]"=w233, "BoolText.TextColor"=w227) -> ()  [unwired: 2 in, 2 out]
          }
          event "Set Path": Value Change {
            n211 = event-data() -> ()  [unwired: 1 in, 1 out]
            n212 = case shown="True" "Set Path" {
              frame False {
              }
              frame True {
                n213 = local read "Next File Name"() -> (w237:path)
                n214 = File Dialog(4:"SpectralRadar Measurement File" ("pattern label"), 5:"Select" ("button label"), 6:"*.srm" ("pattern"), 7:"Select SpectralRadar Measurement" ("Abfrage"), 9:"Measurement" ("Standardname"), 11:w237) -> (1:w235:bool, 3:w236:path)  [unwired: 1 in, 2 out]
                n215 = case shown="False" w235 {
                  tunnel: w236 -> [w245 _]
                  frame False {
                    n216 = Path To String(path=w245) -> (string=w244:string)
                    n217 = call "set Base Filename.vi"("Base"=w244) -> ("error out"=w246:errorcluster)  [unwired: 1 in]
                    n218 = call "get Next Filename.vi"("error in (no error)"=w246) -> ("Next File Name"=→"Next File Name":path)  [unwired: 1 out]
                  }
                  frame True {
                  }
                }
              }
            }
          }
          event Mouse Down; Mouse Up {
            n219 = event-data() -> ()  [unwired: 1 in, 1 out]
            n220 = call "check for Standby.vi"("ResetTimer"=TRUE) -> ()  [unwired: 2 out]
          }
        }
        n221 = local read "QuitApp"() -> (w155:bool)
      }
    }
    frame #4 {
      n222 = local read "Coloring"() -> (w380:refnum<class "Coloring.lvclass">)
      n223 = local read "GalvoControl"() -> (w379:refnum<class "Probe.lvclass">)
      n224 = call "clear Processing.vi"("Processing"=w381) -> ()  [unwired: 6 in, 1 out]
      n225 = call "clear Coloring.vi"("Coloring"=w380) -> ()  [unwired: 6 in, 1 out]
      n226 = call "close Probe.vi"("GalvoControl"=w379) -> ()  [unwired: 6 in, 1 out]
    }
    frame #5 {
      n227 = call "close Device.vi"("OCTDevice"=w383) -> ()  [unwired: 6 in, 1 out]
    }
    frame #6 {
      n228 = local read "AutoSafe"() -> (w384:bool)
      n229 = case shown="True" w384 {
        frame False {
        }
        frame True {
          n230 = local read "Index of Refraction"() -> (w408:dbl)
          n231 = call "get Config Path.vi"() -> ("Path"=w385:path)  [unwired: 1 in, 1 out]
          n232 = local read "Range X [mm]"() -> (w406:dbl)
          n233 = local read "Saturation"() -> (w396:sgl)
          n234 = local read "Brightness"() -> (w393:sgl)
          n235 = local read "Palette"() -> (w398:T2)
          n236 = local read "Columns"() -> (w410:i32)
          n237 = local read "Contrast"() -> (w392:sgl)
          n238 = local read "Window"() -> (w401:T1)
          n239 = Build Path(base path=w385, name or relative path=path "Settings.ini" ("Relative \"SpectralRadar.ini\" Path")) -> (appended path=w412:path)
          n240 = call "init Settings.vi"("Path to settings file"=w412) -> ("Settings"=w405:refnum<class "Settings.lvclass">)  [unwired: 5 in, 1 out]
          n241 = call "set Settings Entry Int.vi"("Value"=w410, "Node"="Columns" ("Node Name"), "Settings"=w405) -> ("Settings"=w404:refnum<class "Settings.lvclass">)  [unwired: 3 in, 1 out]
          n242 = call "set Settings Entry Float.vi"("Value"=w408, "Node"="IndexOfRefraction" ("Node Name"), "Settings"=w404) -> ("Settings"=w403:refnum<class "Settings.lvclass">)  [unwired: 3 in, 1 out]
          n243 = call "set Settings Entry Float.vi"("Value"=w406, "Node"="Range" ("Node Name"), "Settings"=w403) -> ("Settings"=w388:refnum<class "Settings.lvclass">)  [unwired: 3 in, 1 out]
          n244 = call "set Settings Entry Float.vi"("Value"=w396, "Node"="Saturation" ("Node Name"), "Settings"=w388) -> ("Settings"=w395:refnum<class "Settings.lvclass">)  [unwired: 3 in, 1 out]
          n245 = call "set Settings Entry Float.vi"("Value"=w393, "Node"="Brightness" ("Node Name"), "Settings"=w395) -> ("Settings"=w391:refnum<class "Settings.lvclass">)  [unwired: 3 in, 1 out]
          n246 = call "set Settings Entry Float.vi"("Value"=w392, "Node"="Contrast" ("Node Name"), "Settings"=w391) -> ("Settings"=w390:refnum<class "Settings.lvclass">)  [unwired: 3 in, 1 out]
          n247 = call "set Settings Entry Int.vi"("Value"=w401, "Node"="ApodizationWindow" ("Node Name"), "Settings"=w390) -> ("Settings"=w399:refnum<class "Settings.lvclass">)  [unwired: 3 in, 1 out]
          n248 = call "set Settings Entry Int.vi"("Value"=w398, "Node"="Palette" ("Node Name"), "Settings"=w399) -> ("Settings"=w387:refnum<class "Settings.lvclass">)  [unwired: 3 in, 1 out]
          n249 = call "save Settings.vi"("Settings"=w387) -> ("Settings"=w386:refnum<class "Settings.lvclass">)  [unwired: 5 in, 1 out]
          n250 = call "close Settings.vi"("Settings"=w386) -> ()  [unwired: 6 in, 1 out]
        }
      }
    }
  }
